vi "Open and Min WND.vi"(0 "Py Doc in":refnum<class "Py Doc.lvclass">, 5 "Document Path":path, 11 "error in (no error)":errorcluster) -> (4 "Py Editor.lvclass":refnum<class "Py Editor.lvclass">, 6 "Py Shell.lvclass":refnum<class "Py Shell.lvclass">, 15 "error out":errorcluster)   [LabVIEW 2016, in "Py Doc.lvclass"]
uses:
  Py Doc.lvclass
  Child Classes/Py Editor/Py Editor.lvclass
  D:/MDI Project/source code/Document/Py Doc/Py Doc.lvclass
  Child Classes/Py Shell/Py Shell.lvclass
  Py Doc.lvclass/Py Doc.ctl
  Property/Write Py File Path.vi
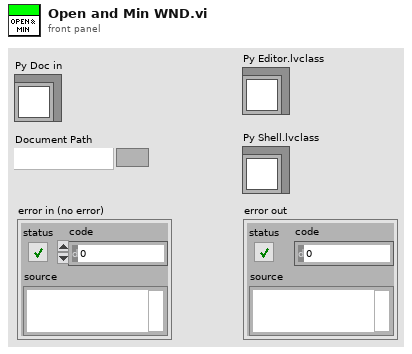
[diagram p1: front panel]
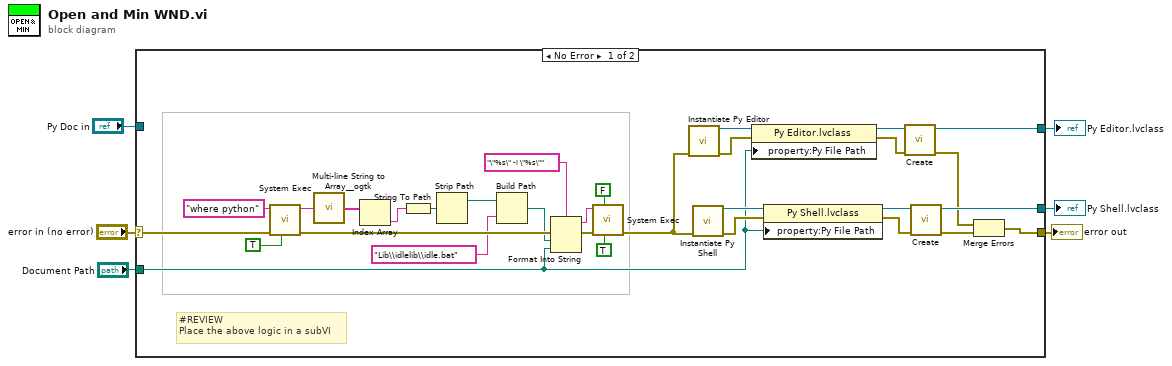
[diagram p0: block diagram]
diagram:
  n1 = case shown="No Error" "error in (no error)" {
    selector: "error in (no error)" -> [w20 w38]
    tunnel: "Py Doc in" -> [_ _]
    tunnel: [w9 w38] -> w5
    tunnel: [w12 _] -> w1
    tunnel: [w10 _] -> w2
    tunnel: "Document Path" -> [w7 _]
    frame No Error {
      # "#REVIEW\nPlace the above logic in a subVI"
      n2 = call <vilib>:"System Exec.vi"("run minimized? (F)"=TRUE, "error in (no error)"=w20, "command line"="where python") -> ("error out"=w37:errorcluster, "standard output"=w25:string)  [unwired: 5 in, 2 out]
      n3 = call <userlib>:"Multi-line String to Array__ogtk.vi"("string"=w25) -> ("lines"=w26:string[])
      n4 = Index Array(array=w26) -> (element=w24:string)  [unwired: 1 in]
      n5 = String To Path(string=w24) -> (path=w33:path)
      n6 = Strip Path(path=w33) -> (stripped path=w34:path)  [unwired: 1 out]
      n7 = Build Path(base path=w34, name or relative path="Lib\\idlelib\\idle.bat") -> (appended path=w36:path)
      n8 = Format Into String(format string="\"%s\" -i \"%s\"", error in=w37, w36, w7) -> (resulting string=w28:string, error out=w27:errorcluster)  [unwired: 1 in]
      n9 = call <vilib>:"System Exec.vi"("run minimized? (F)"=TRUE, "wait until completion? (T)"=FALSE, "error in (no error)"=w27, "command line"=w28) -> ("error out"=w13:errorcluster)  [unwired: 4 in, 3 out]
      n10 = call "Instantiate Py Editor.vi"("error in (no error)"=w13) -> ("Py Editor in"=w18:refnum<class "Py Editor.lvclass">, "error out"=w21:errorcluster)  [unwired: 13 in]
      n11 = call "Instantiate Py Shell.vi"("error in (no error)"=w13) -> ("Py Shell.lvclass"=w15:refnum<class "Py Shell.lvclass">, "error out"=w22:errorcluster)  [unwired: 13 in]
      n12 = property class="Py Editor.lvclass"(reference=w18, error in=w21, "property:Py File Path"=w7) -> (reference out=w17:refnum<class "Py Editor.lvclass">, error out=w19:errorcluster)
      n13 = property class="Py Shell.lvclass"(reference=w15, error in=w22, "property:Py File Path"=w7) -> (reference out=w14:refnum<class "Py Shell.lvclass">, error out=w16:errorcluster)
      n14 = call-dynamic "Create.vi"("error in (no error)"=w19, "Document in"=w17) -> ("error out"=w8:errorcluster, "Document out"=w10:refnum<class "Py Editor.lvclass">)  [unwired: 8 in]
      n15 = call-dynamic "Create.vi"("error in (no error)"=w16, "Document in"=w14) -> ("error out"=w11:errorcluster, "Document out"=w12:refnum<class "Py Shell.lvclass">)  [unwired: 8 in]
      n16 = Merge Errors(w8, w11) -> (w9:errorcluster)
    }
    frame Error {
    }
  }
  "error out" <- w5
  "Py Editor.lvclass" <- w2
  "Py Shell.lvclass" <- w1
